vi "NI VeriStand - Get FIFO Depth.vi"(8 "error in (no error)":errorcluster, 11 "Device Ref in":T1 format="%.0x") -> (0 "error out":errorcluster, 1 "Size FIFO Sink":u32, 2 "Size FIFO Source":u32, 3 "Device Ref out":T1 format="%.0x")   [LabVIEW 2020, in "Custom Device API.lvlib"]
doc: "Returns the depths, or buffer sizes, of the FIFOs of an asynchronous custom device."
uses:
  <vilib>/NI VeriStand/Custom Device API/Custom Device API.lvlib
  <vilib>/NI VeriStand/Custom Device API/Custom Device Item Ref.ctl
  75fd42d8-9fd2-46a4-a470-4bc871284388.vi
  <vilib>/NI VeriStand/Custom Device API/Custom Device Offline Path.vi
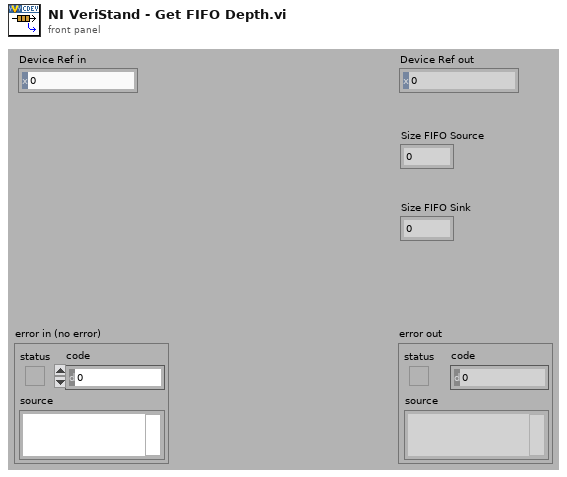
[diagram p1: front panel]
types:
  T1 = typedef "Custom Device API.lvlib/Custom Device Item Ref.ctl" = u64
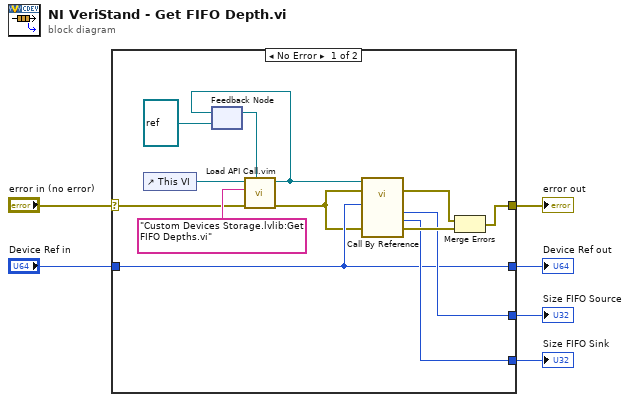
[diagram p0: block diagram]
diagram:
  n1 = case shown="No Error" "error in (no error)" {
    selector: "error in (no error)" -> [w8 w21]
    tunnel: [w18 w21] -> w6
    tunnel: "Device Ref in" -> [w15 w20]
    tunnel: [w15 w20] -> w4
    tunnel: [w17 _] -> w3
    tunnel: [w16 _] -> w2
    frame No Error {
      n2 = control-ref of="This VI"() -> (w10:refnum<vi>)
      n3 = feedback #1(refnum<vi> refnum ("type specifier VI Refnum (for type only)")) -> (w14:refnum<vi>)
      n4 = call "Load API Call.vim"("VI reference in"=w14, "error in (no error)"=w8, "VI qualified name"="Custom Devices Storage.lvlib:Get FIFO Depths.vi", "Caller VI ref"=w10) -> ("error out"=w12:errorcluster, "VI reference"=w13:refnum<vi>)  [unwired: 6 in]
      n5 = feedback-in #1(w13) -> ()
      n6 = call-by-ref "?"(reference=w13, error in=w12, 8:"error in (no error)"=w12, "Device Ref in"=w15) -> (error out=w7:errorcluster, 0:"error out"=w19:errorcluster, "Size FIFO Sink"=w16:u32, "Size FIFO Source"=w17:u32)  [unwired: 6 in, 2 out]
      n7 = Merge Errors(w7, w19) -> (w18:errorcluster)
    }
    frame Error {
    }
  }
  "Device Ref out" <- w4
  "error out" <- w6
  "Size FIFO Source" <- w3
  "Size FIFO Sink" <- w2
